vi "first.vi"() -> ()   [LabVIEW 2012]
panel:
  out "degree":dbl
  in  "radians":dbl
  out "radian":dbl
  in  "degree":dbl
  in  "delay":dbl(slide) scale=0.0..1.0
  out "blink":bool
  in  "stop":bool
  in  "x":dbl(slide) scale=0.0..10.0
  out "2^x":dbl(slide) scale=0.0..1024.0
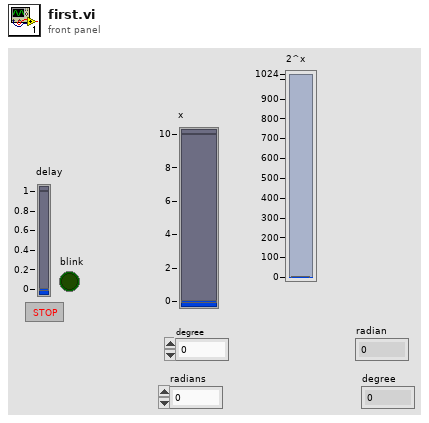
[diagram p1: front panel]
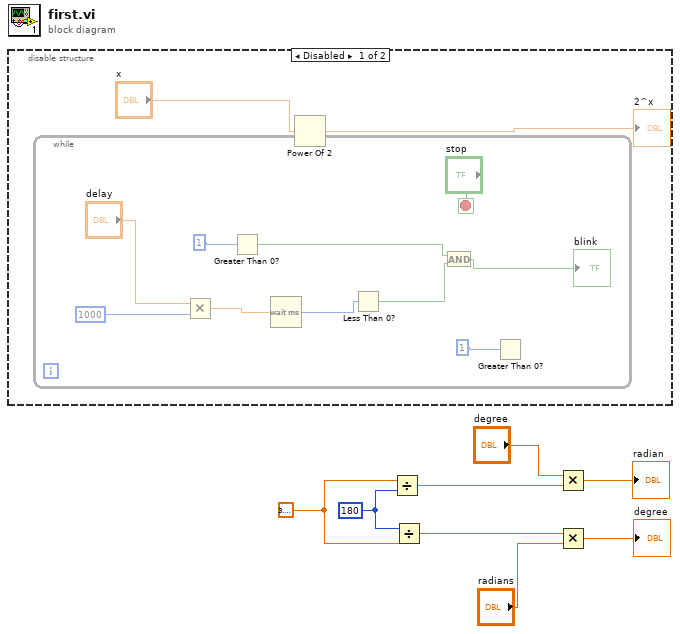
[diagram p0: block diagram]
diagram:
  w5 = 180
  w2 = 3.141592653589793
  n1 = disable-structure shown="Disabled" {
    frame Disabled {
      n2 = while {
        stop <- "stop" stop-if-true
        n3 = Multiply(x="delay", y=1000) -> (x*y=w19:dbl)
        n4 = Greater Than 0?(x=1) -> (x > 0?=w13:bool)
        n5 = Wait (ms)(milliseconds to wait=w19) -> (millisecond timer value=w16:u32)
        n6 = Less Than 0?(x=w16) -> (x < 0?=w15:bool)
        n7 = And(x=w13, y=w15) -> (x .and. y?=→"blink":bool)
        n8 = Greater Than 0?(x=1) -> ()  [unwired: 1 out]
      }
      n9 = Power Of 2(x="x") -> (2^x=→"2^x":dbl)
    }
    frame Enabled {
    }
  }
  n10 = Divide(x=w2, y=w5) -> (x/y=w4:dbl)
  n11 = Divide(x=w5, y=w2) -> (x/y=w3:dbl)
  n12 = Multiply(x="degree", y=w4) -> (x*y=→"radian":dbl)
  n13 = Multiply(x=w3, y="radians") -> (x*y=→"degree":dbl)
